vi "Untitled 2.vi"() -> ()   [LabVIEW 2019, in "lv-apt-json-file-test.lvlib"]
uses:
  lv-apt-json-file-test.lvlib
  <vilib>/JDP Science/JSONtext/JSONtext.lvlib
panel:
  out "<JSON>":string caption="<JSON>First JSON Value"
  out "Rest of Input String":string
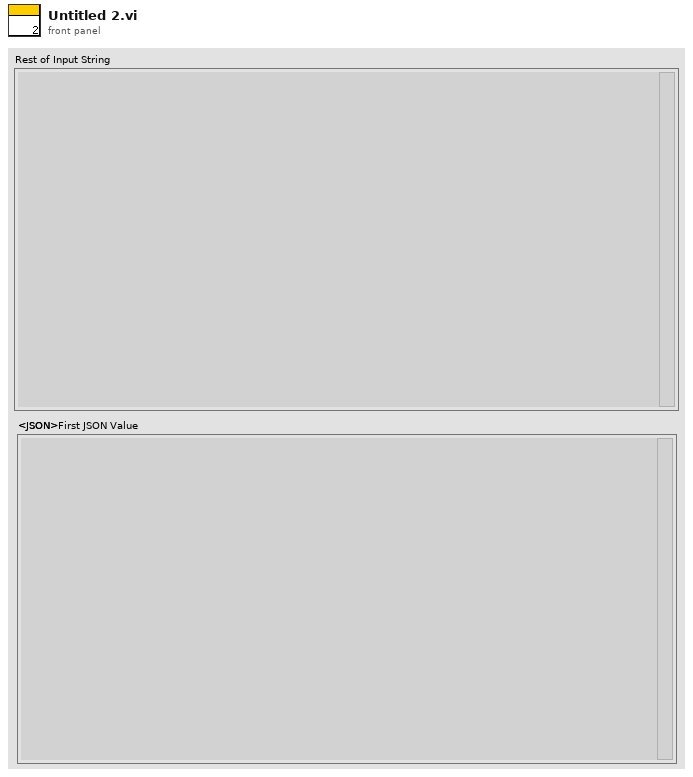
[diagram p1: front panel]
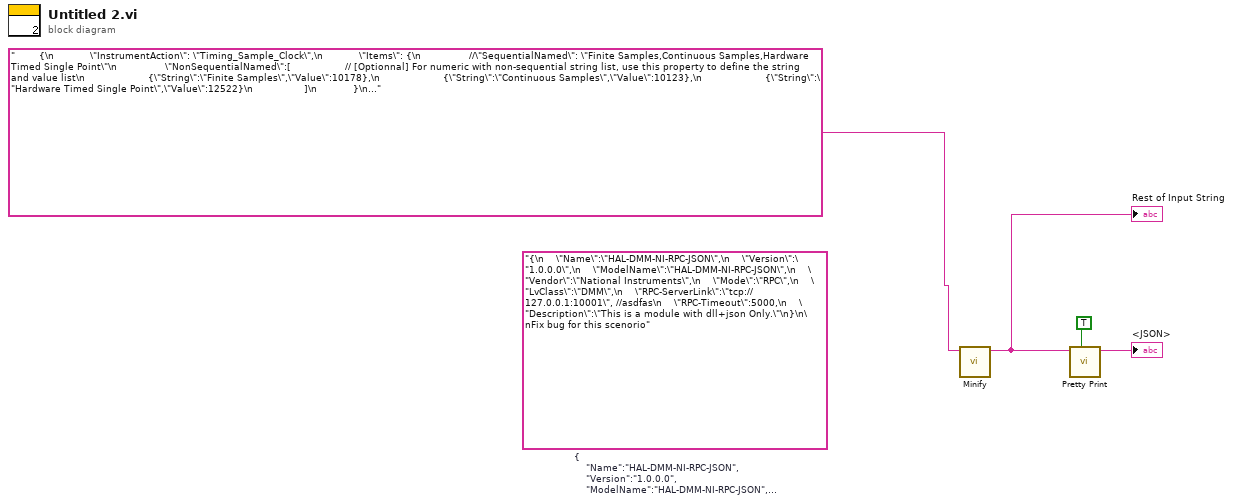
[diagram p0: block diagram]
diagram:
  (unwired) "{\n    \"Name\":\"HAL-DMM-NI-RPC-JSON\",\n    \"Version\":\"1.0.0.0\",\n    \"ModelName\":\"HAL-DMM-NI-RPC-JSON\",\n    \"Vendor\":\"National Instruments\",\n    \"Mode\":\"RPC\",\n    \"LvClass\":\"DMM\",\n    \"RPC-ServerLink\":\"tcp://127.0.0.1:10001\", //asdfas\n    \"RPC-Timeout\":5000,\n    \"Description\":\"This is a module with dll+json Only.\"\n}\n\nFix bug for this scenorio"  # {     "Name":"HAL-DMM-NI-RPC-JSON",     "Version":"1.0.0.0",     "ModelName":"HAL-DMM-NI-RPC-JSON",     "Vendor":"National Instruments",     "Mode":"RPC",     "LvClass":"DMM",     "RPC-ServerLink":"tcp://127.0.0.1:10001", //asdfas     "RPC-Timeout":5000,     "Description":"This is a module with dll+json Only." }  Fix bug for this scenorio
  n1 = call <vilib>:"Minify.vi"("JSON"="        {\n            \"InstrumentAction\": \"Timing_Sample_Clock\",\n            \"Items\": {\n                //\"SequentialNamed\": \"Finite Samples,Continuous Samples,Hardware Timed Single Point\"\n                \"NonSequentialNamed\":[                  // [Optionnal] For numeric with non-sequential string list, use this property to define the string and value list\n                     {\"String\":\"Finite Samples\",\"Value\":10178},\n                     {\"String\":\"Continuous Samples\",\"Value\":10123},\n                     {\"String\":\"Hardware Timed Single Point\",\"Value\":12522}\n                 ]\n            }\n        }") -> ("<JSON>"=w1:string)  [unwired: 8 in, 2 out]
  "Rest of Input String" <- w1
  n2 = call <vilib>:"Pretty Print.vi"("Comment out unparsable lines"=TRUE, "JSON"=w1) -> ("<JSON>"=→"<JSON>":string)  [unwired: 7 in, 2 out]
